vi "Normalized Case Decode.vi"(0 "m":u32[](array[numeric]), 1 "n-m":u32[](array[numeric]), 2 "table":dbl[][](array[numeric]) format="%.2f") -> (3 "m*":u32[](array[numeric]), 4 "n-m*":u32[](array[numeric]), 5 "table*":dbl[][](array[numeric]) format="%.2f", 6 "error":i32)   [LabVIEW 2010, in "NI_Gmath.lvlib"]
uses:
  NI_Gmath.lvlib
panel:
  in  "Case Constant\n(See Context Help)":bool=TRUE
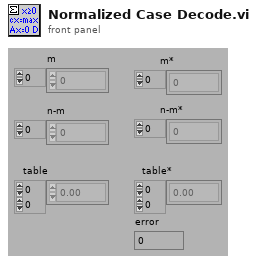
[diagram p1: front panel]
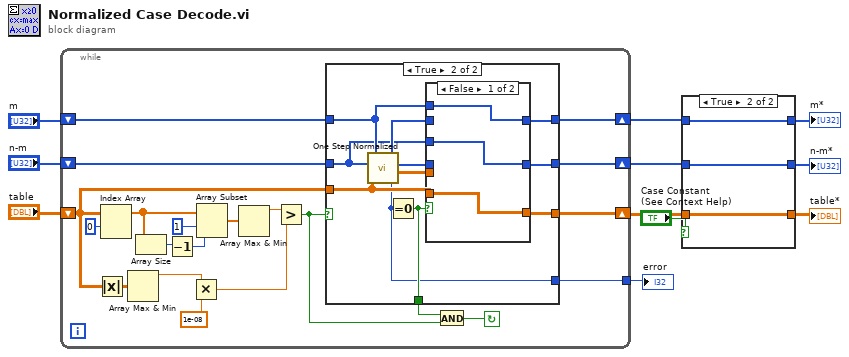
[diagram p0: block diagram]
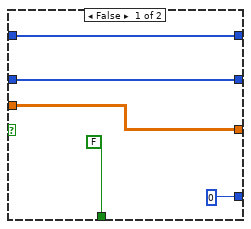
[diagram p2: hidden frame]
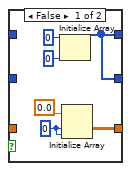
[diagram p4: hidden frame]
diagram:
  n1 = while {
    tunnel: [w18] -> w8
    shift-left: "table" -> [w16]
    shift-right: [w19] -> w7
    shift-left: "n-m" -> [w24]
    shift-right: [w23] -> w6
    shift-left: "m" -> [w26]
    shift-right: [w25] -> w5
    stop <- w20 continue-if-true
    n2 = Absolute Value(x=w16) -> (abs(x)=w15:dbl[][])
    n3 = Index Array(array=w16, index (row)=0) -> (element=w30:dbl[])  [unwired: 1 in]
    n4 = Array Max & Min(array=w15) -> (max value=w14:dbl)  [unwired: 3 out]
    n5 = Array Size(array=w30) -> (size(s)=w29:i32)
    n6 = Decrement(x=w29) -> (x-1=w28:i32)
    n7 = Multiply(x=w14, y=1e-08) -> (x*y=w12:dbl)
    n8 = Array Subset(array=w30, index=1, length=w28) -> (w27:dbl[])
    n9 = Array Max & Min(array=w27) -> (max value=w17:dbl)  [unwired: 3 out]
    n10 = Greater?(x=w17, y=w12) -> (0:w21:bool)
    n11 = case shown="True" w21 {
      tunnel: w26 -> [w37 w42]
      tunnel: [w37 w47] -> w25
      tunnel: w16 -> [w36 w39]
      tunnel: [w36 w43] -> w19
      tunnel: w24 -> [w35 w41]
      tunnel: [w35 w45] -> w23
      tunnel: [FALSE w40] -> w22
      tunnel: [0 w38] -> w18
      frame False {
      }
      frame True {
        n12 = call "One Step Normalized.vi"("m"=w42, "n-m"=w41, "table"=w39) -> ("m*"=w48:u32[], "n-m*"=w46:u32[], "table*"=w44:dbl[][], "error"=w38:i32)
        n13 = Equal To 0?(x=w38) -> (x = 0?=w40:bool)
        n14 = case shown="False" w40 {
          tunnel: w48 -> [_ w54]
          tunnel: [w51 w54] -> w47
          tunnel: w46 -> [_ w53]
          tunnel: [w50 w53] -> w45
          tunnel: w44 -> [_ w52]
          tunnel: [w49 w52] -> w43
          tunnel: w42 -> [w51 _]
          tunnel: w41 -> [w50 _]
          tunnel: w39 -> [w49 _]
          frame False {
          }
          frame True {
          }
        }
      }
    }
    n15 = And(x=w22, y=w21) -> (x .and. y?=w20:bool)
  }
  "error" <- w8
  n16 = case shown="True" "Case Constant\n(See Context Help)" {
    tunnel: w5 -> [_ w63]
    tunnel: [w59 w63] -> w4
    tunnel: w6 -> [_ w62]
    tunnel: [w59 w62] -> w3
    tunnel: [w55 w61] -> w2
    tunnel: w7 -> [_ w61]
    frame False {
      w57 = 0
      n17 = Initialize Array(u32 0, 0) -> (w59:u32[])
      n18 = Initialize Array(0.0, w57, w57) -> (w55:dbl[][])
    }
    frame True {
    }
  }
  "n-m*" <- w3
  "m*" <- w4
  "table*" <- w2
